vi "Log Entry to Timestamp.vi"(8 "error in (no error)":errorcluster, 11 "String":string) -> (0 "error out":errorcluster, 3 "Time Stamp":timestamp)   [LabVIEW 2019]
doc: "Convert a log entry's time stamp into a LabVIEW timestamp"
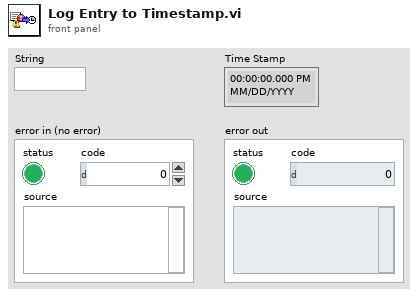
[diagram p1: front panel]
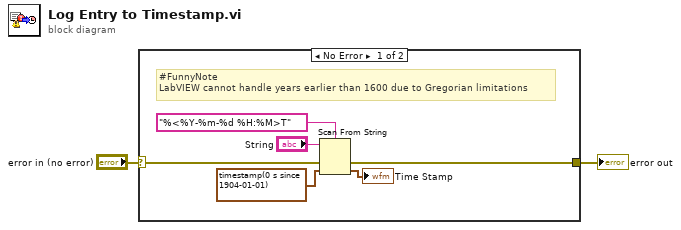
[diagram p0: block diagram]
diagram:
  n1 = case shown="No Error" "error in (no error)" {
    selector: "error in (no error)" -> [w3 w9]
    tunnel: [w7 w9] -> w2
    frame No Error {
      # "#FunnyNote\nLabVIEW cannot handle years earlier than 1600 due to Gregorian limitations"
      n2 = Scan From String(format string="%<%Y-%m-%d %H:%M>T", input string="String", error in=w3, default 1=timestamp(0 s since 1904-01-01) ("Time Stamp")) -> (error out=w7:errorcluster, output 1=→"Time Stamp":timestamp)  [unwired: 1 in, 2 out]
    }
    frame Error {
    }
  }
  "error out" <- w2
